vi "GetErrorsOfLibrary.vi"(8 "ErrorIn":errorcluster caption="Error In(no Error)", 9 "LibraryName":string, 10 "ErrorCodes":i32[](array[numeric]), 11 "ReferenceIn":refnum<class "ErrorDefinitionSQLite.lvclass"> caption="Reference In") -> (0 "ErrorOut":errorcluster caption="Error Out", 1 "Errors":T1[](array[typedef]), 3 "ReferenceOut":refnum<class "ErrorDefinitionSQLite.lvclass"> caption="Reference Out")   [LabVIEW 2021, in "ErrorDefinitionSQLite.lvclass"]
uses:
  ErrorDefinitionSQLite.lvclass
  <vilib>/drjdpowell/SQLite Library/SQLite.lvlib
  ErrorContent.ctl
  _CreateCustomErrorWithDataConfig.llb/Flag.ctl
  <vilib>/drjdpowell/SQLite Library/SQL Connection/Execute SQL.vi
  <vilib>/drjdpowell/SQLite Library/SQL Connection/Connection.lvclass
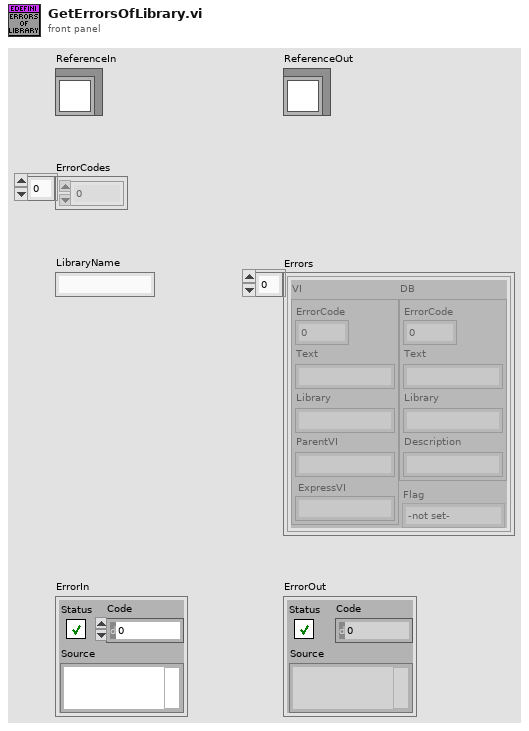
[diagram p1: front panel]
types:
  T1 = typedef "ErrorDefinitionSQLite.lvclass/ErrorContent.ctl" = cluster{"VI":cluster{"ErrorCode":i32, "Text":string, "Library":string, "ParentVI":string, "ExpressVI":string}, "DB":cluster{"ErrorCode":i32, "Text":string, "Library":string, "Description":string}, "Flag":T2}
  T2 = typedef "Flag.ctl" = enum16{"-not set-", "OK", "DB Only", "VI Only", "Text Mismatch", "Library Mismatch", "Different Error", "Updated", "New Error Code", "Add Existing Error Code", "Delete Entry", "New Error Code This VI"}
  T3 = typedef "ErrorDefinitionSQLite.lvclass/ObjectAttributes.ctl" = cluster{"Path":path, "SQLiteRef":refnum<class "Connection.lvclass">, "EndOfRange":i32, "StartOfRange":i32}
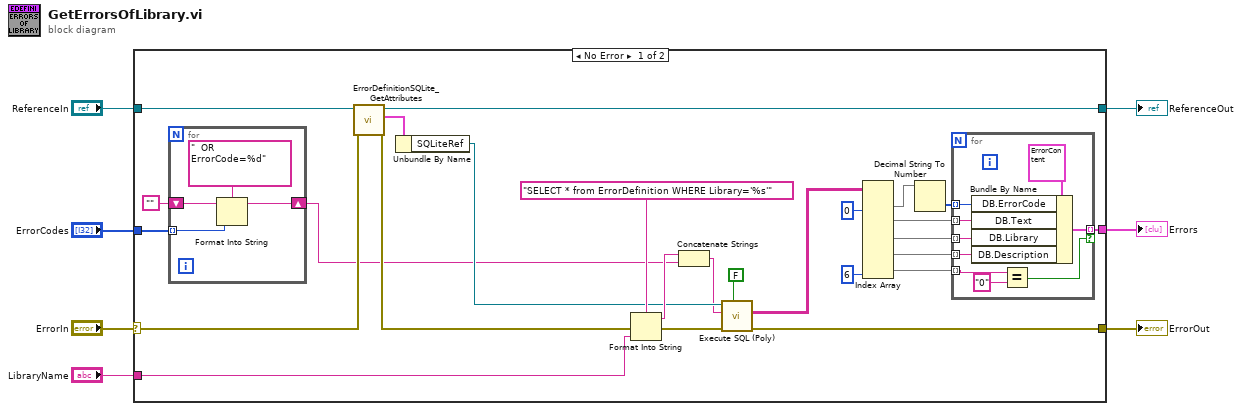
[diagram p0: block diagram]
diagram:
  n1 = case shown="No Error" "ErrorIn" {
    selector: "ErrorIn" -> [w33 w48]
    tunnel: [w30 w48] -> w6
    tunnel: [w28 w47] -> w4
    tunnel: "ReferenceIn" -> [w29 w47]
    tunnel: "LibraryName" -> [w23 _]
    tunnel: [w15 _] -> w2
    tunnel: "ErrorCodes" -> [w13 _]
    frame No Error {
      n2 = for {
        tunnel: w13 -> [w35] mode=indexing
        shift-right: [w36] -> w8
        shift-left: "" -> [w37]
        n3 = Format Into String(format string="  OR ErrorCode=%d", initial string=w37, w35) -> (resulting string=w36:string)  [unwired: 1 in, 1 out]
      }
      n4 = call "ErrorDefinitionSQLite_GetAttributes.vi"("ErrorIn"=w33, "ReferenceIn"=w29) -> ("ErrorOut"=w31:errorcluster, "Data"=w27:T3, "ReferenceOut"=w28:refnum<class "ErrorDefinitionSQLite.lvclass">)  [unwired: 6 in, 1 out]
      n5 = Unbundle By Name(w27) -> ("SQLiteRef"=w14:refnum<class "Connection.lvclass">)
      n6 = Format Into String(format string="SELECT * from ErrorDefinition WHERE Library='%s'" ("SQL"), error in=w31, w23) -> (resulting string=w24:string, error out=w32:errorcluster)  [unwired: 1 in]
      n7 = Concatenate Strings(w24, w8) -> (w11:string)
      n8 = call-poly <vilib>:"Execute SQL (Poly).vi"("Use SAVEPOINT"=FALSE, "error in (no error)"=w32, "SQL"=w11, "SQLite Connection in"=w14) -> ("error out"=w30:errorcluster, "Result Set"=w22:string[][])  [unwired: 4 in, 2 out]
      n9 = Index Array(array=w22, index (col) #1=0 ("disabled index (col)"), index (col) #5=6 ("index (col)")) -> (element #1=w17:string[], element #2=w18:string[], element #3=w19:string[], element #4=w20:string[], element #5=w10:string[])  [unwired: 8 in]
      n10 = Decimal String To Number(string=w17) -> (number=w16:i32[])  [unwired: 2 in, 1 out]
      n11 = for {
        tunnel: w20 -> [w45] mode=indexing
        tunnel: w19 -> [w44] mode=indexing
        tunnel: w18 -> [w43] mode=indexing
        tunnel: w16 -> [w42] mode=indexing
        tunnel: [w41] -> w15 mode=indexing if=w38
        tunnel: w10 -> [w40] mode=indexing
        n12 = Bundle By Name(cluster=T1 {"VI"={"ErrorCode"=0, "Text"="", "Library"="", "ParentVI"="", "ExpressVI"=""}, "DB"={"ErrorCode"=0, "Text"="", "Library"="", "Description"=""}, "Flag"=enum."-not set-"} ("Errors"), "DB.ErrorCode"=w42, "DB.Text"=w43, "DB.Library"=w44, "DB.Description"=w45) -> (w41:T1)
        n13 = Equal?(x=w40, y="0") -> (x = y?=w38:bool)
      }
    }
    frame Error {
    }
  }
  "ErrorOut" <- w6
  "ReferenceOut" <- w4
  "Errors" <- w2
